vi "fgv_lane_slope-info.vi"(7 "cmd":enum16{"ini", "read", "write"}(ring), 8 "error in":errorcluster, 11 "diff slope":dbl) -> (0 "error out":errorcluster, 2 "lane cross":bool, 3 "diff slope out":dbl)   [LabVIEW 2019]
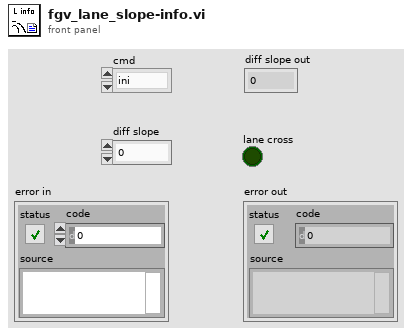
[diagram p1: front panel]
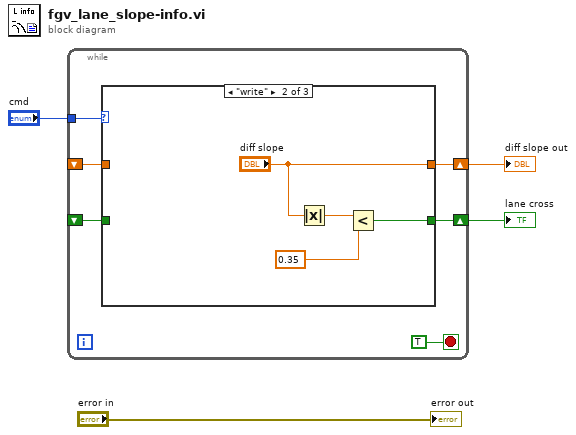
[diagram p0: block diagram]
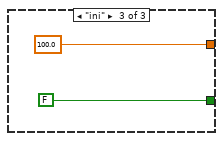
[diagram p3: hidden frame]
diagram:
  n1 = while {
    tunnel: "cmd" -> [w9]
    shift-right: [w8] -> w2
    shift-left: _ -> [w7]
    shift-right: [w6] -> w1
    shift-left: _ -> [w5]
    stop <- TRUE stop-if-true
    n2 = case shown="\"write\"" w9 {
      tunnel: [w12 "diff slope" 100.0 ("diff slope")] -> w8
      tunnel: w7 -> [w12 _ _]
      tunnel: [w11 w13 FALSE] -> w6
      tunnel: w5 -> [w11 _ _]
      frame "read", Default {
      }
      frame "write" {
        n3 = Absolute Value(x="diff slope") -> (abs(x)=w15:dbl)
        n4 = Less?(x=w15, y=0.35) -> (x < y?=w13:bool)
      }
      frame "ini" {
      }
    }
  }
  "diff slope out" <- w2
  "lane cross" <- w1
  "error out" <- "error in"
